vi "ManipChangeGoalTargetPosition.vi"(10 "Instruction String":string) -> (1 "Error Out":errorcluster, 2 "Advance Trigger":bool)   [LabVIEW 2020]
uses:
  SafeParser_Float.vi
  autonomousinfo.vi
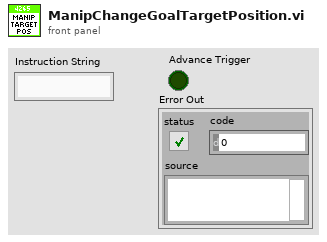
[diagram p1: front panel]
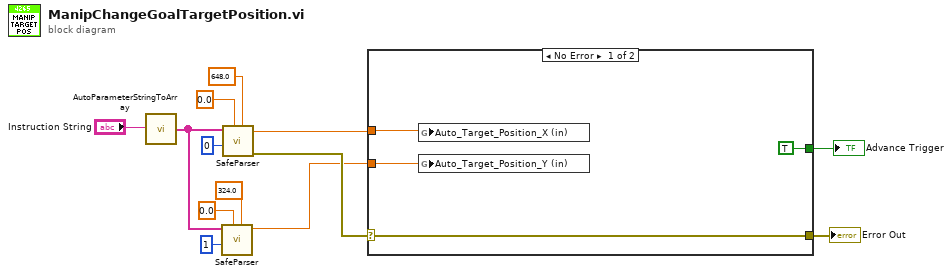
[diagram p0: block diagram]
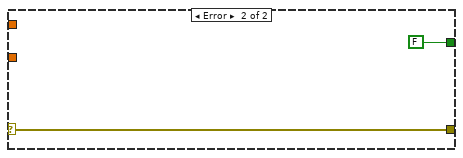
[diagram p2: hidden frame]
diagram:
  n1 = call "AutoParameterStringToArray.vi"("Parameter String"="Instruction String") -> ("Parsed Parameters"=w5:string[])
  n2 = call-poly "SafeParser.vi"("Maximum"=324.0, "Minimum"=0.0, "Array Index"=1, "String Array"=w5) -> ("Typecast  Value"=w1:dbl)  [unwired: 6 in, 1 out]
  n3 = call-poly "SafeParser.vi"("Maximum"=648.0, "Minimum"=0.0, "Array Index"=0 ("Parameter Index"), "String Array"=w5) -> ("Error Out"=w12:errorcluster, "Typecast  Value"=w13:dbl)  [unwired: 6 in]
  n4 = case shown="No Error" w12 {
    selector: w12 -> [w16 w18]
    tunnel: [TRUE ("Advance Trigger") FALSE ("Advance Trigger")] -> w10
    tunnel: [w16 w18] -> w9
    tunnel: w13 -> [w15 _]
    tunnel: w1 -> [w14 _]
    frame No Error {
      n5 = global write "autonomousinfo.vi" "Auto_Target_Position_X (in)"(w15) -> ()
      n6 = global write "autonomousinfo.vi" "Auto_Target_Position_Y (in)"(w14) -> ()
    }
    frame Error {
    }
  }
  "Advance Trigger" <- w10
  "Error Out" <- w9
